vi "Short Name to Path (Unicode).vi"(8 "error in":errorcluster, 11 "LabVIEW Path":path) -> (0 "error out":errorcluster, 3 "UTF-8 Path":refnum<class "UTF-8 Path.lvclass">)   [LabVIEW 2020, in "G-Unicode.lvlib"]
doc: "Converts the LabVIEW path in 8.3 short name format to the corresponding unicode path. Note that the path must exist on disk.\n\n<b>Windows only.</b> Linux and macOS will return a UTF-8 encoded path."
uses:
  G-Unicode.lvlib
  Types/UTF-8 Path/UTF-8 Path.lvclass
  Types/UTF-8 Path/UTF-8 Path.lvclass/UTF-8 Path.ctl
  Private/Memory/Copy String.vi
  Private/Library/Result To Error.vi
  Private/Memory/Copy String.vi/4d47babd-4a2d-4eb7-b91b-7e707d692665.vi
  Private/Library/gu_free.vi
  <vilib>/Utility/error.llb/Error Cluster From Error Code.vi
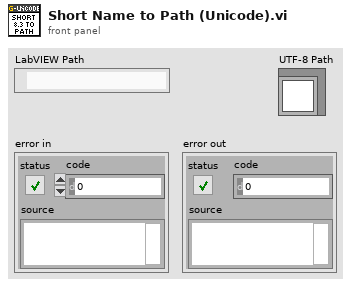
[diagram p1: front panel]
types:
  T1 = typedef "G-Unicode.lvlib/Encoded UTF-8 String.ctl" = string
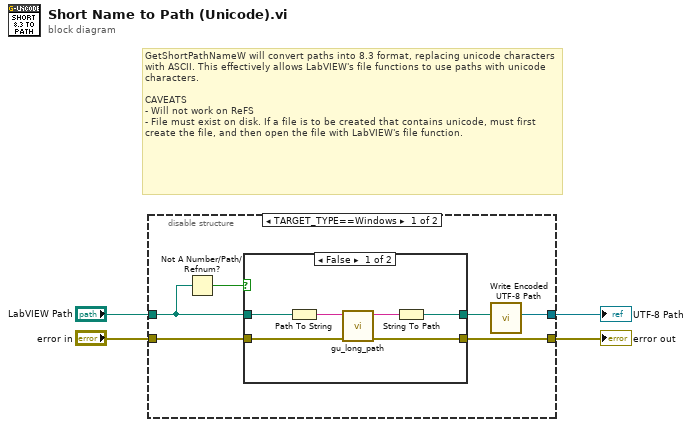
[diagram p0: block diagram]
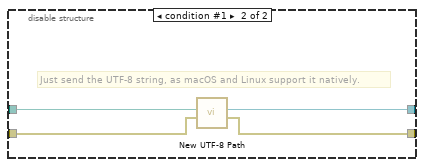
[diagram p3: hidden frame]
diagram:
  # "GetShortPathNameW will convert paths into 8.3 format, replacing unicode characters with ASCII. This effectively allows LabVIEW's file functions to use paths with unicode characters.\n\nCAVEATS\n- Will not work on ReFS\n- File must exist on disk. If a file is to be created that contains unicode, must first create the file, and then open the file with LabVIEW's file function."
  n1 = disable-structure shown="TARGET_TYPE==Windows" {
    disable-tunnel: [w5 w19] -> w1
    disable-tunnel: "LabVIEW Path" -> [w8 w20]
    disable-tunnel: "error in" -> [w9 w21]
    disable-tunnel: [w10 w22] -> w3
    frame condition #0 (active) {
      n2 = Not A Number/Path/Refnum?(number/path/refnum=w8) -> (NaN/Path/Refnum?=w7:bool)
      n3 = case shown="False" w7 {
        tunnel: [w11 w17] -> w10
        tunnel: w8 -> [w16 w18]
        tunnel: w9 -> [w12 w17]
        tunnel: [w13 w18] -> w6
        frame False {
          n4 = Path To String(path=w16) -> (string=w15:string)
          n5 = call "gu_long_path.vi"("error in"=w12, "Path"=w15) -> ("error out"=w11:errorcluster, "Long Path"=w14:T1)  [unwired: 8 in]
          n6 = String To Path(string=w14) -> (path=w13:path)
        }
        frame True {
        }
      }
      n7 = call "Write Encoded UTF-8 Path.vi"("Encoded UTF-8 Path"=w6) -> ("UTF-8 Path"=w5:refnum<class "UTF-8 Path.lvclass">)  [unwired: 10 in]
    }
    frame condition #1 {
      # "Just send the UTF-8 string, as macOS and Linux support it natively."
      n8 = call "New UTF-8 Path.vi"("error in"=w21, "LabVIEW Path"=w20) -> ("error out"=w22:errorcluster, "UTF-8 Path"=w19:refnum<class "UTF-8 Path.lvclass">)  [unwired: 8 in]
    }
  }
  "error out" <- w3
  "UTF-8 Path" <- w1
